vi "Open FPGA V5.2 Unified.vi"() -> (0 "error out":errorcluster, 1 "SlaveRef":T1, 2 "Master Ref":T2, 3 "P2P ref":refnum<k20>)   [LabVIEW 2015]
uses:
  Controls/FpgaMasterRef Typedef.ctl
  Controls/FpgaSlaveRef Unified Typedef.ctl
  <vilib>/FPGAPlugInAG/PXIe-7962R/niLvFpga_Open_PXIe-7962R.vi
  <vilib>/FPGAPlugInAG/PXIe-7962R/niLvFpga_Abort_PXIe-7962R.vi
  <vilib>/rvi/interface/common/niFpgaWaitOnOcc.vi
  <vilib>/Utility/error.llb/Error Cluster From Error Code.vi
  <vilib>/FPGAPlugInAG/PXIe-7962R/niLvFpga_Run_PXIe-7962R.vi
  <vilib>/rvi/interface/nirviOpenFPGA/nirviOpenFPGA.xnode
  FPGA Bitfiles/GMLIDARV5.1_FPGATarget_LIDAR5.1UnifiedV_TptdWXfnG2s.lvbitx
  FPGA/LIDAR 5.1 Unified Version V1.vi
  <vilib>/rvi/interface/nirviMethod/nirviMethod.xnode
  <vilib>/rvi/errors/niLvFpgaMergeErrorWithErrorCode.vi
  <vilib>/rvi/interface/nirviReadWriteControl/nirviReadWriteControl.xnode
  <vilib>/FPGAPlugInAG/PXIe-7972R/niLvFpga_Open_PXIe-7972R.vi
  <vilib>/FPGAPlugInAG/PXIe-7972R/niLvFpga_Abort_PXIe-7972R.vi
  <vilib>/FPGAPlugInAG/PXIe-7972R/niLvFpga_P2PGetEndpoint_PXIe-7972R.vi
  NiFpgaLv.dll
  <vilib>/rvi/errors/niLvFpgaAdjustHostInterfaceError.vi
  <vilib>/FPGAPlugInAG/PXIe-7972R/niLvFpga_Run_PXIe-7972R.vi
  FPGA Bitfiles/LidarMasterV5.2.1.lvbitx
  <vilib>/FPGAPlugInAG/PXIe-7962R/niLvFpga_ConfigureFifo_PXIe-7962R.vi
  <vilib>/FPGAPlugInAG/PXIe-7962R/niLvFpga_StartFifo_PXIe-7962R.vi
  <vilib>/FPGAPlugInAG/PXIe-7962R/niLvFpga_P2PGetEndpoint_PXIe-7962R.vi
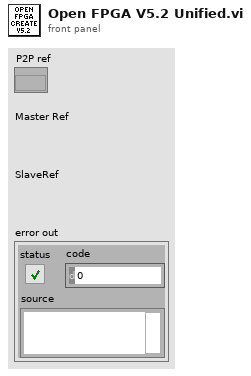
[diagram p1: front panel]
types:
  T1 = typedef "FpgaSlaveRef Unified Typedef.ctl" = refnum<k20>
  T2 = typedef "FpgaMasterRef Typedef.ctl" = refnum<k20>
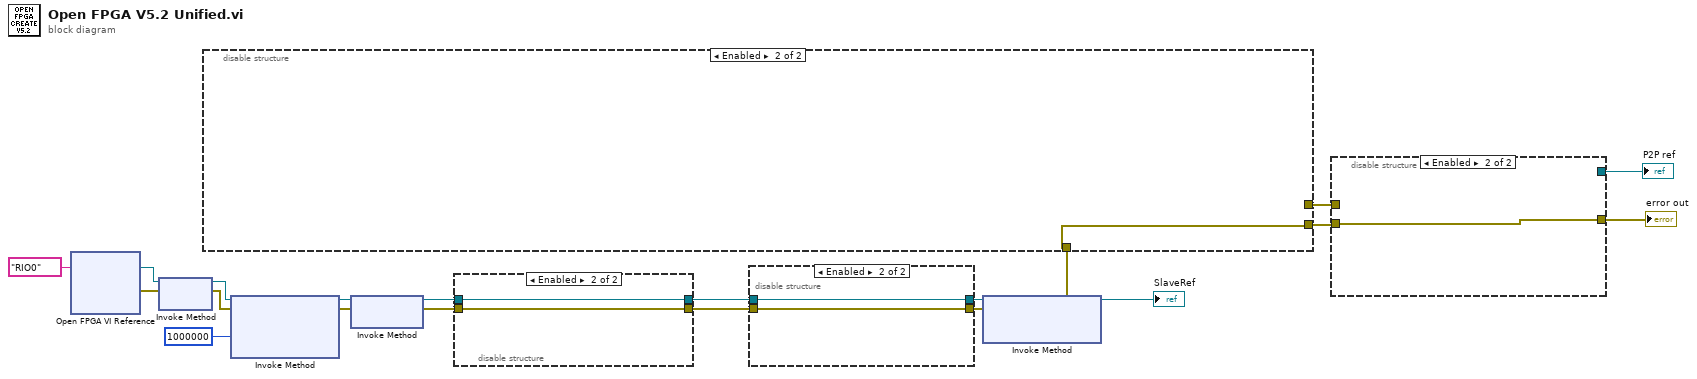
[diagram p0: block diagram]
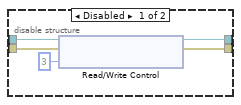
[diagram p2: hidden frame]
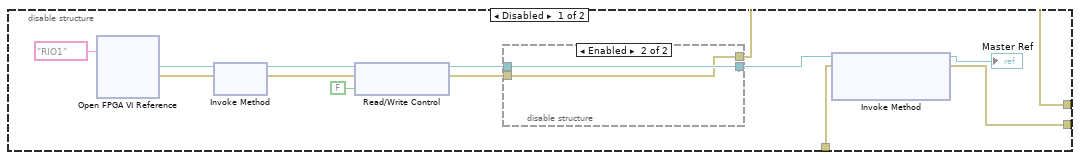
[diagram p3: hidden frame]
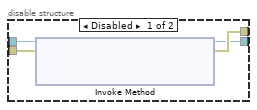
[diagram p4: hidden frame]
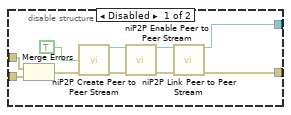
[diagram p5: hidden frame]
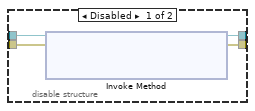
[diagram p6: hidden frame]
diagram:
  n1 = xnode "Open FPGA VI Reference"("resource name"=tag "RIO0") -> ("FPGA VI Reference Out"=w12:T1, "error out"=w13:errorcluster)  [unwired: 1 in]
  n2 = xnode "Invoke Method"("FPGA VI Reference In"=w12, "error in"=w13) -> ("FPGA VI Reference Out"=w14:T1, "error out"=w16:errorcluster)
  n3 = xnode "Invoke Method"("FPGA VI Reference In"=w14, "error in"=w16, "Requested Depth"=u32 1000000) -> ("FPGA VI Reference Out"=w17:T1, "error out"=w18:errorcluster)  [unwired: 1 out]
  n4 = xnode "Invoke Method"("FPGA VI Reference In"=w17, "error in"=w18) -> ("FPGA VI Reference Out"=w19:T1, "error out"=w20:errorcluster)
  n5 = disable-structure shown="Enabled" {
    disable-tunnel: w20 -> [w25 w26]
    disable-tunnel: w19 -> [w24 w27]
    disable-tunnel: [w22 w27] -> w6
    disable-tunnel: [w21 w26] -> w4
    frame Disabled {
      n6 = xnode "Invoke Method"("FPGA VI Reference In"=w24, "error in"=w25) -> ("FPGA VI Reference Out"=w22:T1, "error out"=w21:errorcluster, "Reader"=w23)
    }
    frame Enabled {
    }
  }
  n7 = disable-structure shown="Enabled" {
    disable-tunnel: w6 -> [w32 w34]
    disable-tunnel: [w30 w34] -> w5
    disable-tunnel: w4 -> [w29 w33]
    disable-tunnel: [w28 w33] -> w3
    frame Disabled {
      n8 = xnode "Read/Write Control"("FPGA VI Reference In"=w32, "error in"=w29, "Sample Clock Select"=u8 3) -> ("FPGA VI Reference Out"=w30:T1, "error out"=w28:errorcluster)
    }
    frame Enabled {
    }
  }
  n9 = xnode "Invoke Method"("FPGA VI Reference In"=w5, "error in"=w3) -> ("FPGA VI Reference Out"=→"SlaveRef":T1, "error out"=w8:errorcluster)  [unwired: 1 in]
  n10 = disable-structure shown="Enabled" {
    disable-tunnel: [w47 _] -> w11
    disable-tunnel: [w46 w55] -> w10
    disable-tunnel: w8 -> [w44 w55]
    frame Disabled {
      n11 = xnode "Open FPGA VI Reference"("resource name"=tag "RIO1") -> ("FPGA VI Reference Out"=w41:T2, "error out"=w42:errorcluster)  [unwired: 1 in]
      n12 = xnode "Invoke Method"("FPGA VI Reference In"=w41, "error in"=w42) -> ("FPGA VI Reference Out"=w39:T2, "error out"=w37:errorcluster)
      n13 = xnode "Read/Write Control"("FPGA VI Reference In"=w39, "error in"=w37, "StartSyncLoop"=FALSE) -> ("FPGA VI Reference Out"=w38:T2, "error out"=w36:errorcluster)
      n14 = disable-structure shown="Enabled" {
        disable-tunnel: w36 -> [w52 w53]
        disable-tunnel: w38 -> [w51 w54]
        disable-tunnel: [w50 w53] -> w47
        disable-tunnel: [w49 w54] -> w43
        frame Disabled {
          n15 = xnode "Invoke Method"("FPGA VI Reference In"=w51, "error in"=w52) -> ("FPGA VI Reference Out"=w49:T2, "error out"=w50:errorcluster, "Writer"=w48)
        }
        frame Enabled {
        }
      }
      n16 = xnode "Invoke Method"("FPGA VI Reference In"=w43, "error in"=w44) -> ("FPGA VI Reference Out"=→"Master Ref":T2, "error out"=w46:errorcluster)  [unwired: 1 in]
    }
    frame Enabled {
    }
  }
  n17 = disable-structure shown="Enabled" {
    disable-tunnel: w11 -> [w67 _]
    disable-tunnel: w10 -> [w66 w68]
    disable-tunnel: [w64 w68] -> w9
    disable-tunnel: [w63 _] -> w7
    frame Disabled {
      n18 = Merge Errors(w67, w66) -> (w65:errorcluster)
      n19 = call <vilib>:"niP2P Create Peer to Peer Stream.vi"("enable stream (T)"=TRUE, "error in (no error)"=w65) -> ("writer"=w56:refnum<k20>, "stream session"=w59:refnum<k20>, "reader"=w57:refnum<k20>, "error out"=w60:errorcluster)  [unwired: 10 in]
      n20 = call <vilib>:"niP2P Enable Peer to Peer Stream.vi"("stream session"=w59, "error in (no error)"=w60) -> ("stream session out"=w61:refnum<k20>, "error out"=w62:errorcluster)  [unwired: 12 in]
      n21 = call <vilib>:"niP2P Link Peer to Peer Stream.vi"("stream session"=w61, "error in (no error)"=w62) -> ("stream session out"=w63:refnum<k20>, "error out"=w64:errorcluster)  [unwired: 12 in]
    }
    frame Enabled {
    }
  }
  "error out" <- w9
  "P2P ref" <- w7
